vi "StringMergerProj2.vi"(0 "FilterType":string, 1 "Aproximace":string, 2 "Rad":dbl, 3 "Nizka frekvence":dbl, 4 "Vysoka frekvence":dbl, 5 "Username":string, 6 "Min Frequency":dbl, 7 "Max Frequency":dbl, 9 "Step":dbl, 11 "Fmez":dbl) -> (20 "Output string":string)   [LabVIEW 2021]
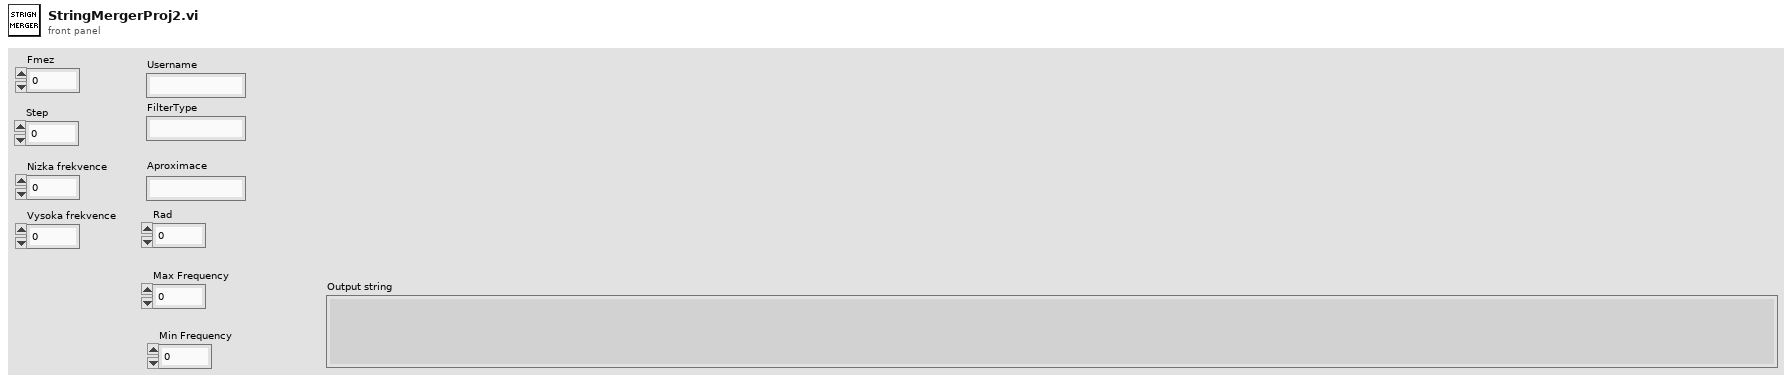
[diagram p1: front panel]
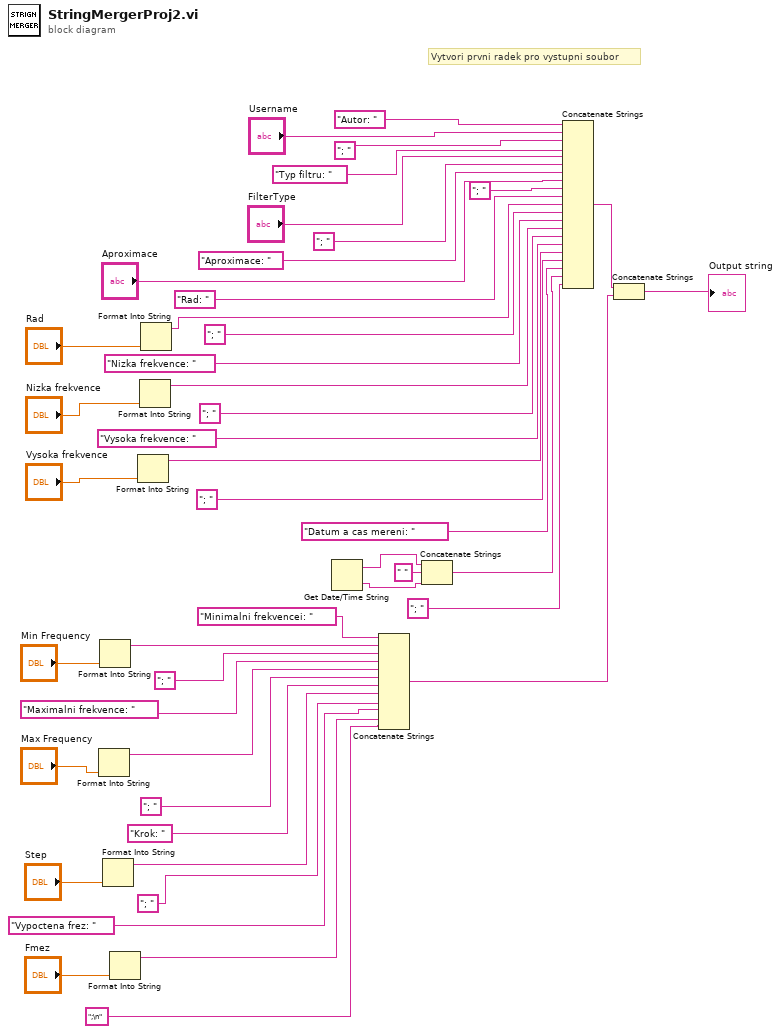
[diagram p0: block diagram]
diagram:
  # "Vytvori prvni radek pro vystupni soubor"
  n1 = Format Into String("Max Frequency") -> (resulting string=w25:string)  [unwired: 3 in, 1 out]
  n2 = Format Into String("Min Frequency") -> (resulting string=w28:string)  [unwired: 3 in, 1 out]
  n3 = Format Into String("Step") -> (resulting string=w23:string)  [unwired: 3 in, 1 out]
  n4 = Format Into String("Fmez") -> (resulting string=w19:string)  [unwired: 3 in, 1 out]
  n5 = Format Into String("Vysoka frekvence") -> (resulting string=w5:string)  [unwired: 3 in, 1 out]
  n6 = Format Into String("Nizka frekvence") -> (resulting string=w9:string)  [unwired: 3 in, 1 out]
  n7 = Format Into String("Rad") -> (resulting string=w13:string)  [unwired: 3 in, 1 out]
  n8 = Get Date/Time String() -> (date string=w39:string, time string=w38:string)  [unwired: 3 in]
  n9 = Concatenate Strings("Minimalni frekvencei: " ("string"), w28, "; " ("string"), "Maximalni frekvence: " ("string"), w25, "; " ("string"), "Krok: " ("string"), w23, "; " ("string"), "Vypoctena frez: " ("string"), w19, ";\n" ("string")) -> (w31:string)
  n10 = Concatenate Strings(w39, " " ("string"), w38) -> (w2:string)
  n11 = Concatenate Strings("Autor: " ("string"), "Username", "; " ("string"), "Typ filtru: " ("string"), "FilterType", "; " ("string"), "Aproximace: " ("string"), "Aproximace", "; " ("string"), "Rad: " ("string"), w13, "; " ("string"), "Nizka frekvence: " ("string"), w9, "; " ("string"), "Vysoka frekvence: " ("string"), w5, "; " ("string"), "Datum a cas mereni: " ("string"), w2, "; " ("string")) -> (w30:string)
  n12 = Concatenate Strings(w30, w31) -> (→"Output string":string)
